vi "Builder.vi"(3 "error in (no error)":errorcluster, 4 "Clear Cards":bool=TRUE, 5 "Array IN":i32[](array[numeric])) -> (0 "error out (no error)":errorcluster)   [LabVIEW 2011]
uses:
  Server_Globals.vi
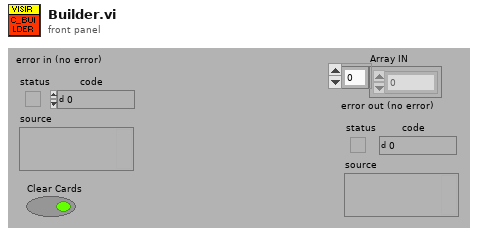
[diagram p1: front panel]
types:
  T1 = cluster{"I/O Settings":u64[], "Instrument Handle":cluster{"5402":refnum<k15>, " 5112":refnum<k15>, "4072":refnum<k15>, "USB":refnum<visa-resource-name>, "4110":refnum<k15>}, "Logfile":refnum<file>, "Log Level":i8, "Clear":i32[], "OS Set":cluster{"instrument handle out":refnum<k15>, "remaining string":string, "Settings":cluster{"Horizontal Conf.":cluster{"Min. Sample rate":dbl, "Reference position":dbl, "Record Length":i16}, "Channel A":cluster{"Enable":bool, "Vertical coupling":dbl, "Vertical range":dbl, "Vertical offset":dbl, "Probe attenuation":dbl}, "Channel B":cluster{"Enable":bool, "Vertical coupling":dbl, "Vertical range":dbl, "Vertical offset":dbl, "Probe attenuation":dbl}, "Trigger":cluster{"Source":enum8{"channel 1", "channel 2", "Imediate", "External trigger"}, "Slope":enum8{"Positive", "Negative"}, "Coupling":enum8{"AC", "DC"}, "Level":dbl, "Holdoff":dbl, "Delay":dbl, " Timeout":dbl, " Mode":enum8{"Normal", "Auto", "Auto Level"}}, "Measurements":cluster{"Measurement 1, Channel":enum8{"Channel 1", "Channel 2", "Channel 3", "Channel 4"}, "Measurement 1, Selection":u16, "Measurement 2, Channel":enum8{"Channel 1", "Channel 2", "Channel 3", "Channel 4"}, "Measurement 2,  Selection":u16, "Measurement 3, Channel":enum8{"Channel 1", "Channel 2", "Channel 3", "Channel 4"}, "Measurement 3, Selection 3":u16}}}, "DC Power Supply":cluster{"0":refnum<k15>, "1":refnum<k15>, "2":refnum<k15>, "3":refnum<k15>, "4":refnum<k15>}, "USB Interface":cluster{"0":refnum<visa-resource-name>, "1":refnum<visa-resource-name>, "2":refnum<visa-resource-name>, "3":refnum<visa-resource-name>, "4":refnum<visa-resource-name>}, "Function Generator":cluster{"0":refnum<k15>, "1":refnum<k15>, "2":refnum<k15>, "3":refnum<k15>, "4":refnum<k15>}, "Digital Multimeter":cluster{"0":refnum<k15>, "1":refnum<k15>, "2":refnum<k15>, "3":refnum<k15>, "4":refnum<k15>}, "Digital Osciliscope":cluster{"0":refnum<k15>, "1":refnum<k15>, "2":refnum<k15>, "3":refnum<k15>, "4":refnum<k15>}, "To M Server":string, "Adres":string[][], "Matrix version":string, "MD5":string, "Digital Multimeter Card 2":cluster{"0":string, "1":string, "2":string, "3":string, "4":string}}
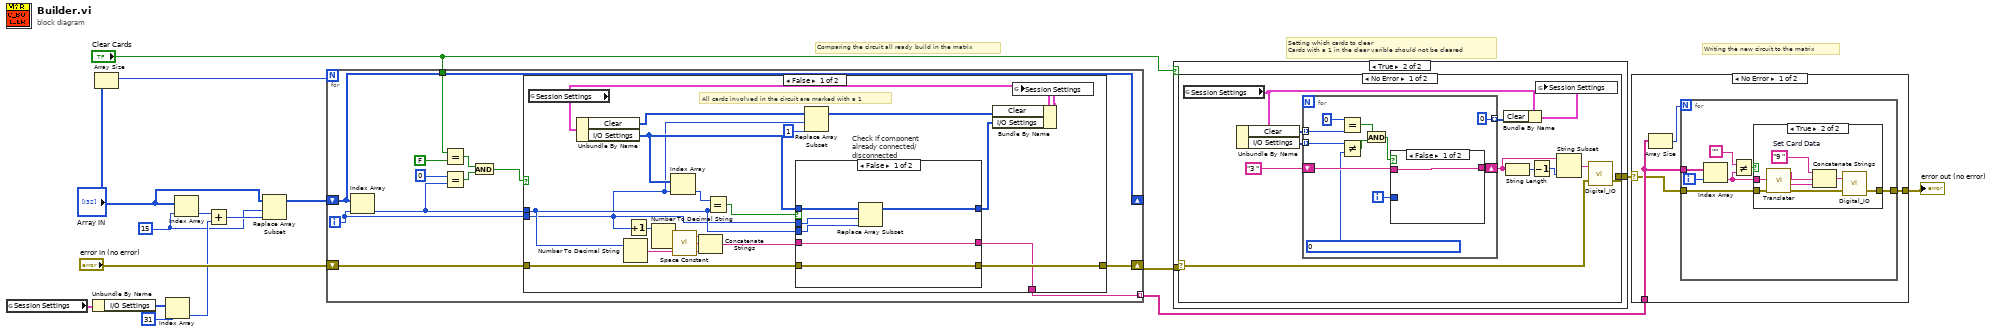
[diagram p0: block diagram]
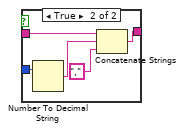
[diagram p3: hidden frame]
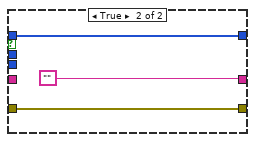
[diagram p7: hidden frame]
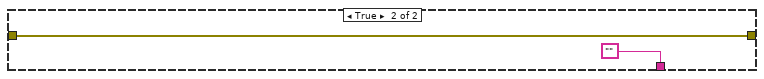
[diagram p8: hidden frame]
diagram:
  w1 = 15
  # "Writing the new circuit to the matrix"
  # "Setting which cards to clear\nCards with a 1 in the clear varible should not be cleared"
  # "Comparing the circuit all ready build in the matrix"
  n1 = global read "Server_Globals.vi" "Session Settings"() -> (w9:T1)
  n2 = Unbundle By Name(w9) -> ("I/O Settings"=w8:u64[])
  n3 = Array Size(array="Array IN") -> (size(s)=w15:i32)
  n4 = Index Array(array=w8, index=31) -> (element=w5:u64)
  n5 = Index Array(array="Array IN", index=w1) -> (element=w6:i32)
  n6 = Add(x=w6, y=w5) -> (x+y=w4:u64)
  n7 = Replace Array Subset(array="Array IN", new element=w4, index=w1) -> (w2:i32[])
  n8 = for {
    N: w15 -> [_]
    shift-right: [w27] -> w16
    shift-left: "error in (no error)" -> [w28]
    tunnel: [w26] -> w14 mode=indexing
    shift-right: [w25] -> _
    shift-left: w2 -> [w25]
    tunnel: "Clear Cards" -> [w21]
    i -> [w24]
    n9 = Index Array(array=w25, index=w24) -> (element=w23:i32)
    n10 = Equal?(x=w21, y=FALSE) -> (x = y?=w18:bool)
    n11 = Equal?(x=0, y=w23) -> (x = y?=w19:bool)
    n12 = And(x=w18, y=w19) -> (x .and. y?=w17:bool)
    n13 = case shown="False" w17 {
      tunnel: w28 -> [w44 w58]
      tunnel: [w43 w58] -> w27
      tunnel: [w36 ""] -> w26
      tunnel: w23 -> [w33 _]
      tunnel: w24 -> [w29 _]
      frame False {
        # "All cards involved in the circuit are marked with a 1"
        n14 = global read "Server_Globals.vi" "Session Settings"() -> (w42:T1)
        n15 = Unbundle By Name(w42) -> ("Clear"=w37:i32[], "I/O Settings"=w38:u64[])
        n16 = Number To Decimal String(number=w33) -> (decimal integer string=w32:string)  [unwired: 1 in]
        n17 = Increment(x=w29) -> (x+1=w30:i32)
        n18 = Number To Decimal String(number=w30) -> (decimal integer string=w34:string)  [unwired: 1 in]
        n19 = Index Array(array=w38, index=w29) -> (element=w46:u64)
        n20 = call <vilib>:"Space Constant.vi"() -> ("String"=w35:string)
        n21 = Concatenate Strings(w34, w35, w32) -> (w31:string)
        n22 = Equal?(x=w46, y=w33) -> (x = y?=w45:bool)
        n23 = case "Check if component already connected/disconnected" shown="False" w45 {
          tunnel: w38 -> [w52 w56]
          tunnel: [w53 w56] -> w39
          tunnel: w33 -> [w50 _]
          tunnel: w29 -> [w51 _]
          tunnel: w44 -> [w49 w55]
          tunnel: [w49 w55] -> w43
          tunnel: [w48 ""] -> w36
          tunnel: w31 -> [w48 _]
          frame False {
            n24 = Replace Array Subset(array=w52, new element=w50, index=w51) -> (w53:u64[])
          }
          frame True {
          }
        }
        n25 = Replace Array Subset(array=w37, new element=1, index=w29) -> (w40:i32[])
        n26 = Bundle By Name(cluster=w42, "Clear"=w40, "I/O Settings"=w39) -> (w47:T1)
        n27 = global write "Server_Globals.vi" "Session Settings"(w47) -> ()
      }
      frame True {
      }
    }
  }
  n28 = case shown="True" "Clear Cards" {
    tunnel: w16 -> [w59 w61]
    tunnel: [w59 w60] -> w13
    frame False {
    }
    frame True {
      n29 = case shown="No Error" w61 {
        selector: w61 -> [w70 w91]
        tunnel: [w69 w91] -> w60
        frame No Error {
          n30 = global read "Server_Globals.vi" "Session Settings"() -> (w72:T1)
          n31 = Unbundle By Name(w72) -> ("Clear"=w68:i32[], "I/O Settings"=w62:u64[])
          n32 = for {
            tunnel: w68 -> [w83] mode=indexing
            shift-right: [w80] -> w65
            shift-left: "3 " -> [w81]
            tunnel: [0] -> w71 mode=indexing
            tunnel: w62 -> [w77] mode=indexing
            i -> [w82]
            n33 = Equal?(x=0, y=w83) -> (x = y?=w75:bool)
            n34 = Not Equal?(x=w77, y=0) -> (x != y?=w76:bool)
            n35 = And(x=w75, y=w76) -> (x .and. y?=w74:bool)
            n36 = case shown="False" w74 {
              tunnel: w82 -> [_ w88]
              tunnel: w81 -> [w85 w90]
              tunnel: [w85 w89] -> w80
              frame False {
              }
              frame True {
                n37 = Number To Decimal String(number=w88) -> (decimal integer string=w87:string)  [unwired: 1 in]
                n38 = Concatenate Strings(w90, w87, ",") -> (w89:string)
              }
            }
          }
          n39 = Bundle By Name(cluster=w72, "Clear"=w71) -> (w73:T1)
          n40 = String Length(string=w65) -> (length=w64:i32)
          n41 = Decrement(x=w64) -> (x-1=w63:i32)
          n42 = global write "Server_Globals.vi" "Session Settings"(w73) -> ()
          n43 = String Subset(string=w65, length (rest)=w63) -> (substring=w66:string)  [unwired: 1 in]
          n44 = call "Digital_IO.vi"("error in"=w70, "Data in"=w66) -> ("error out (no error)"=w69:errorcluster)  [unwired: 1 in]
        }
        frame Error {
        }
      }
    }
  }
  n45 = case shown="No Error" w13 {
    selector: w13 -> [w92 w112]
    tunnel: w14 -> [w94 _]
    tunnel: [w93 w112] -> w11
    frame No Error {
      n46 = Array Size(array=w94) -> (size(s)=w95:i32)
      n47 = for {
        N: w95 -> [_]
        tunnel: w94 -> [w102]
        tunnel: [w101] -> w93
        tunnel: w92 -> [w100]
        i -> [w99]
        n48 = Index Array(array=w102, index=w99) -> (element=w97:string)
        n49 = Not Equal?(x="", y=w97) -> (x != y?=w98:bool)
        n50 = case shown="True" w98 {
          tunnel: w97 -> [_ w107]
          tunnel: [w103 w106] -> w101
          tunnel: w100 -> [w103 w105]
          frame False {
          }
          frame True {
            w111 = "9 "  # Set Card Data
            n51 = call "Translater.vi"("In"=w107, "error in (no error)"=w105) -> ("Card"=w109:string, "Comp"=w108:string, "error out (no error)"=w104:errorcluster)  [unwired: 2 in]
            n52 = Concatenate Strings(w111, w109, w108) -> (w110:string)
            n53 = call "Digital_IO.vi"("error in"=w104, "Data in"=w110) -> ("error out (no error)"=w106:errorcluster)  [unwired: 1 in]
          }
        }
      }
    }
    frame Error {
    }
  }
  "error out (no error)" <- w11
